vi "ti2_getCustomZSpeed.vi"(8 "error in (no error)":errorcluster) -> (0 "error out":errorcluster, 3 "pUserOutParam":i32[](array[numeric]))   [LabVIEW 2018, in "ti2lv.lvlib"]
uses:
  ti2lv.lvlib
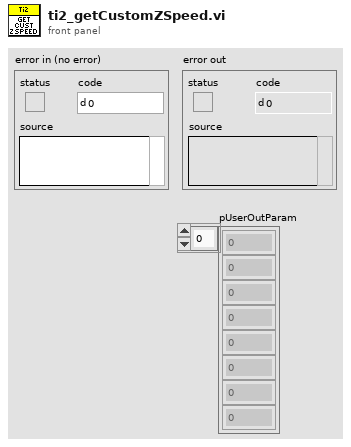
[diagram p1: front panel]
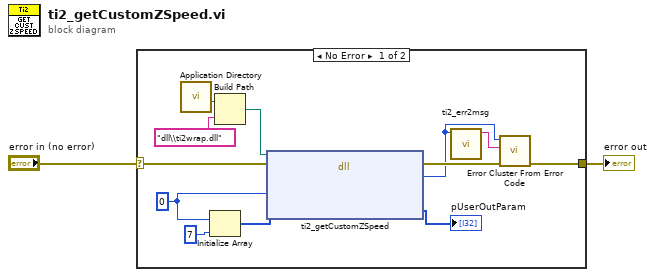
[diagram p0: block diagram]
diagram:
  n1 = case shown="No Error" "error in (no error)" {
    selector: "error in (no error)" -> [w13 w15]
    tunnel: [w14 w15] -> w1
    frame No Error {
      w9 = 0 ("filterPos")
      n2 = call <vilib>:"Application Directory.vi"() -> ("Application Directory"=w4:path)
      n3 = Initialize Array(w9, 7 ("dimension size")) -> (w7:i32[])
      n4 = Build Path(base path=w4, name or relative path="dll\\ti2wrap.dll") -> (appended path=w3:path)
      n5 = dll-call lib="?" fn="ti2_getCustomZSpeed"(path in=w3, error in=w13, "tableNumber"=w9, "pUserOutParam"=w7) -> (error out=w12:errorcluster, "return type"=w11:i32, "pUserOutParam"=→"pUserOutParam":i32[])  [unwired: 2 in, 1 out]
      n6 = call "ti2_err2msg.vi"("Error Code"=w11) -> ("Error Message"=w10:string)  [unwired: 10 in]
      n7 = call <vilib>:"Error Cluster From Error Code.vi"("error in (no error)"=w12, "error message (\"\")"=w10, "error code (0)"=w11) -> ("error out"=w14:errorcluster)  [unwired: 6 in]
    }
    frame Error {
    }
  }
  "error out" <- w1
